vi "Bandlimited Signal Generation.vi"() -> ()   [LabVIEW 2020]
doc: "Demonstrates how to generate a bandlimited signal with the Multitone Generator VI, then calculate its harmonics with the FFT Spectrum (Mag-Phase) VI."
uses:
  <vilib>/Analysis/4window.llb/windowTd.ctl
  <vilib>/Analysis/1siggen.llb/Ramp Pattern by Samples.vi
  <vilib>/measure/maspectr.llb/FFT Spectrum (Mag-Phase) for 1 Chan.vi
  <vilib>/measure/NI_MAPro.lvlib
  <vilib>/Analysis/NI_AALBase.lvlib
  <vilib>/Analysis/NI_AALPro.lvlib
panel:
  in  "Amplitude":dbl=1.0
  in  "Frequency":dbl=3.0
  out "Time Waveform":waveform(dbl)(graph)
  out "largest harmonic":dbl=45.0 format="%#.6g"
  out "# harmonics":dbl=8.0
  out "Magnitude":cluster{"f0":dbl, "df":dbl, "magnitude":dbl[]}(graph)
  # "Overview: Demonstrates how to generate a bandlimited signal.\nRequirements: LabVIEW Full Development System\nInstructions:\nRun the VI. Observe the original Time Waveform, and the Magnitude plot displaying the harmonics that result from performing an FFT on the signal."
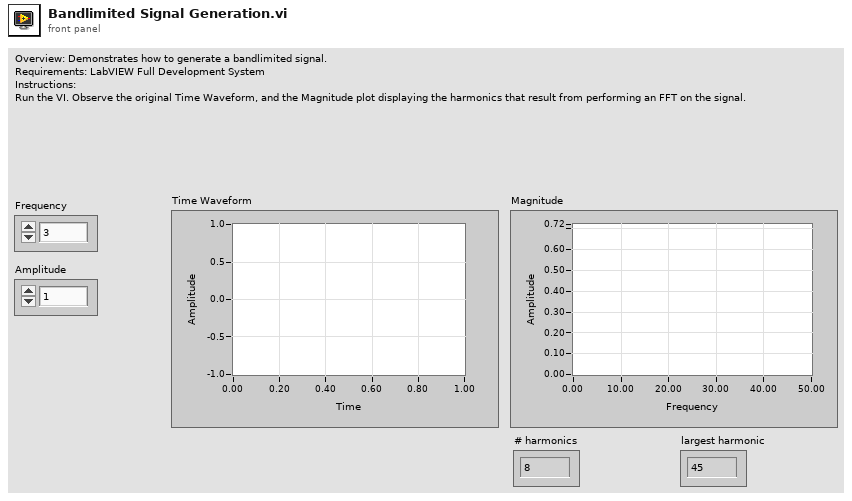
[diagram p1: front panel]
types:
  T1 = typedef "NI_AALPro.lvlib/windowTd.ctl" = u32
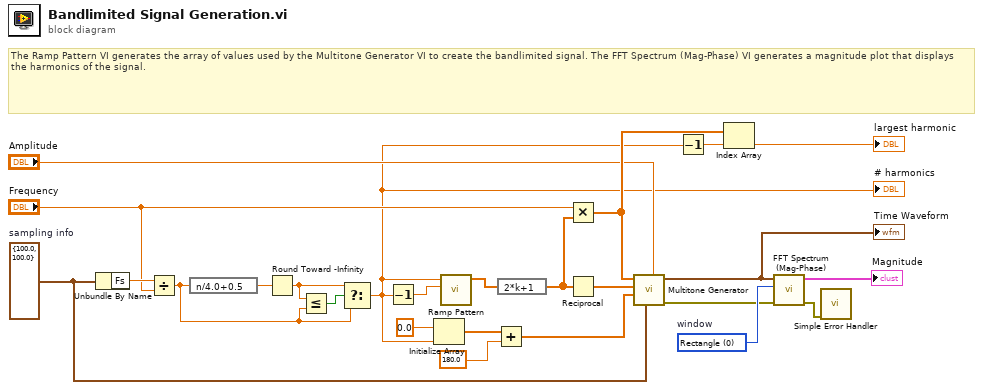
[diagram p0: block diagram]
diagram:
  w10 = T1 0 items=["Rectangle"=0, "Hanning"=1, "Hamming"=2, "Blackman-Harris"=3, "Exact Blackman"=4, "Blackman"=5, "Flat Top"=6, "4 Term B-Harris "=7, "7 Term B-Harris"=8, "Low Sidelobe"=9, "Blackman Nuttall"=11, "Triangle"=30, "Bartlett-Hanning"=31, "Bohman"=32, "Parzen"=33, "Welch"=34, "Kaiser"=60, "Dolph-Chebyshev"=61, "Gaussian"=62]  # window
  w13 = cluster{"Fs":dbl, "#s":dbl} {"Fs"=100.0, "#s"=100.0}  # sampling info
  # "The Ramp Pattern VI generates the array of values used by the Multitone Generator VI to create the bandlimited signal. The FFT Spectrum (Mag-Phase) VI generates a magnitude plot that displays the harmonics of the signal."
  n1 = Unbundle By Name(w13) -> ("Fs"=w21:dbl)
  n2 = Divide(x=w21, y="Frequency") -> (x/y=w12:dbl)
  n3 = expression code="n/4.0+0.5"(w12) -> (w15:dbl)
  n4 = Round Toward -Infinity(1:w15) -> (0:w14:dbl)
  n5 = Less Or Equal?(x=w14, y=w12) -> (x <= y?=w17:bool)
  n6 = Select(t=w14, s=w17, f=w12) -> (s? t:f=w2:dbl)
  "# harmonics" <- w2
  n7 = Decrement(x=w2) -> (x-1=w16:dbl)
  n8 = Initialize Array(0.0, w2) -> (w3:dbl[])
  n9 = call-poly <vilib>:"Ramp Pattern.vi"("end"=w16, "samples"=w2) -> ("Ramp Pattern"=w19:dbl[])  [unwired: 8 in, 1 out]
  n10 = Add(x=w3, y=180.0) -> (x+y=w20:dbl[])
  n11 = expression code="2*k+1"(w19) -> (w18:dbl[])
  n12 = Multiply(x="Frequency", y=w18) -> (x*y=w24:dbl[])
  n13 = Reciprocal(x=w18) -> (1/x=w25:dbl[])
  n14 = call <vilib>:"Multitone Generator.vi"("amplitude"="Amplitude", "sampling info"=w13, "tone phases"=w20, "tone amplitudes"=w25, "tone frequencies"=w24) -> ("error out"=w9:errorcluster, "signal out"=w11:waveform(dbl))  [unwired: 3 in, 2 out]
  "Time Waveform" <- w11
  n15 = Decrement(x=w2) -> (x-1=w23:dbl)
  n16 = Index Array(array=w24, index=w23) -> (element=→"largest harmonic":dbl)
  n17 = call-poly <vilib>:"FFT Spectrum (Mag-Phase).vi"("error in (no error)"=w9, "window"=w10, "time signal"=w11) -> ("error out"=w8:errorcluster, "magnitude"=→"Magnitude":cluster{"f0":dbl, "df":dbl, "magnitude":dbl[]})  [unwired: 4 in, 3 out]
  n18 = call <vilib>:"Simple Error Handler.vi"("error in (no error)"=w8) -> ()  [unwired: 4 in, 5 out]
